vi "Start Autofocus.vi"(11 "RS232":refnum<visa-resource-name>="ASRL27::INSTR") -> (0 "Success?":bool, 3 "RS232 out":refnum<visa-resource-name>="ASRL27::INSTR")   [LabVIEW 2022 SP3]
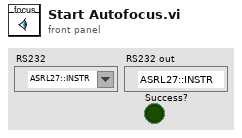
[diagram p1: front panel]
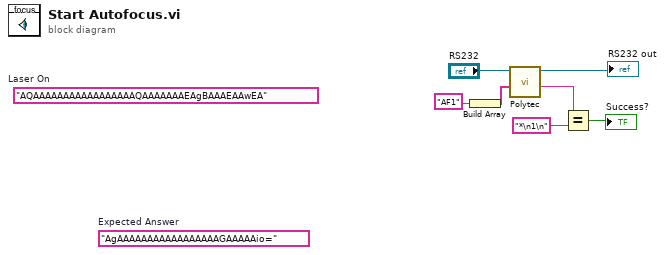
[diagram p0: block diagram]
diagram:
  (unwired) "AQAAAAAAAAAAAAAAAAAQAAAAAAAEAgBAAAEAAwEA"  # Laser On
  (unwired) "AgAAAAAAAAAAAAAAAAAGAAAAAio="  # Expected Answer
  n1 = Build Array("AF1" ("write buffer")) -> (w1:string[])
  n2 = call "Polytec.vi"("RS232"="RS232", "Strings"=w1) -> ("RS232 out"=→"RS232 out":refnum<visa-resource-name>, "String Read"=w4:string)  [unwired: 7 in]
  n3 = Equal?(x=w4, y="*\n1\n") -> (x = y?=→"Success?":bool)
